vi "tutorial-062_ToDLAY.vi"(10 "Control Array":refnum<vi>[](array[refnum]), 11 "Changed Names":string[](array[string])) -> ()   [LabVIEW 2019]
uses:
  TextControlledInstrum/TextControlledInstrum.lvlib
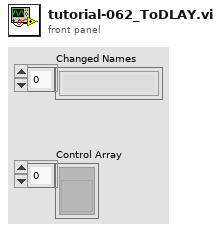
[diagram p1: front panel]
types:
  T1 = cluster{"[0]":string, "[1]":string, "[2]":string}
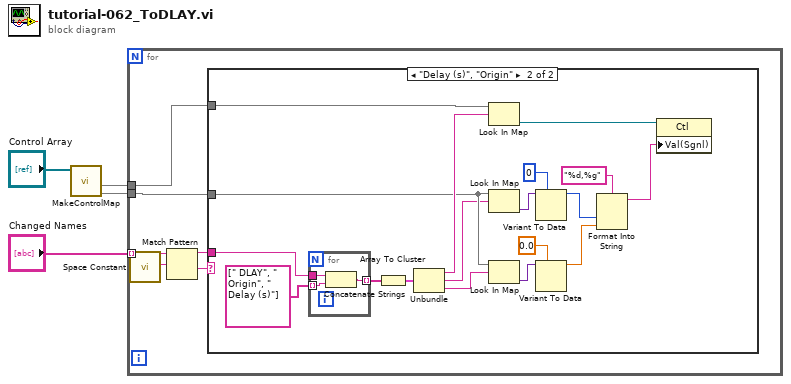
[diagram p0: block diagram]
diagram:
  n1 = call "MakeControlMap.vi"("ControlArray"="Control Array") -> ("ValueMap out"=w1:map{string, variant}, "ControlMap out"=w2:map{string, refnum<vi>})  [unwired: 7 in, 2 out]
  n2 = for {
    tunnel: "Changed Names" -> [w10] mode=indexing
    tunnel: w2 -> [w6]
    tunnel: w1 -> [w5]
    n3 = call <vilib>:"Space Constant.vi"() -> ("String"=w9:string)
    n4 = Match Pattern(string=w10, regular expression=w9) -> (before substring=w7:string, after substring=w8:string)  [unwired: 1 in, 2 out]
    n5 = case shown="\"Delay (s)\", \"Origin\"" w8 {
      tunnel: w7 -> [_ w28]
      tunnel: w6 -> [_ w24]
      tunnel: w5 -> [_ w22]
      frame Default {
      }
      frame "Delay (s)", "Origin" {
        n6 = for {
          tunnel: w28 -> [w31]
          tunnel: string[] [" DLAY", " Origin", " Delay (s)"] -> [w30] mode=indexing
          tunnel: [w29] -> w26 mode=indexing
          n7 = Concatenate Strings(w31, w30) -> (w29:string)
        }
        n8 = Array To Cluster(array=w26) -> (cluster=w25:T1)
        n9 = Unbundle(w25) -> ("[0]"=w23:string, "[1]"=w21:string, "[2]"=w20:string)
        n10 = Look In Map(map=w24, key=w23) -> (value=w12:refnum<vi>)  [unwired: 1 in, 1 out]
        n11 = Look In Map(map=w22, key=w21) -> (value=w19:variant)  [unwired: 1 in, 1 out]
        n12 = Look In Map(map=w22, key=w20) -> (value=w18:variant)  [unwired: 1 in, 1 out]
        n13 = Variant To Data(type=u32 0, Variant=w19) -> (data=w14:u32)  [unwired: 1 in, 1 out]
        n14 = Variant To Data(type=0.0, Variant=w18) -> (data=w15:dbl)  [unwired: 1 in, 1 out]
        n15 = Format Into String(format string="%d,%g", w14, w15) -> (resulting string=w11:string)  [unwired: 2 in, 1 out]
        n16 = property class="Ctl"(reference=w12, "Val(Sgnl)"=w11) -> ()  [unwired: 1 in, 2 out]
      }
    }
  }
